vi "I2C Open.vi"(7 "I2C Channel (0)":u8, 8 "Error In":errorcluster, 11 "LINX Resource":T1) -> (0 "Error Out":errorcluster, 3 "LINX Resource":T1)   [LabVIEW 2011, in "LVH-LINX.lvlib"]
doc: "Open the specified I2C channel."
uses:
  LVH-LINX.lvlib
  Private/Type Defs/LINX Ref.ctl
  Private/Type Defs/Platform.ctl
  Private/Type Defs/Interface.ctl
  Private/Device/Type Defs/LINX Device Config.ctl
  Private/Device/Type Defs/TCP Config.ctl
  Private/Device/Type Defs/Channels.ctl
  Private/Type Defs/Peripheral.ctl
  Private/Type Defs/Channel FGV States.ctl
  Private/Device/Device.lvlib
  Private/myRIO/myRIO.lvlib
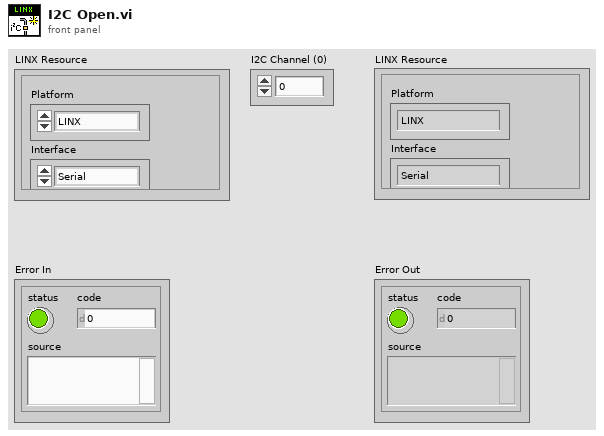
[diagram p1: front panel]
types:
  T1 = typedef "LVH-LINX.lvlib/LINX Ref.ctl" = cluster{"Platform":T2, "Interface":T3, "LINX Device Config":T4}
  T2 = typedef "LVH-LINX.lvlib/Platform.ctl" = enum16{"LINX", "myRIO"}
  T3 = typedef "LVH-LINX.lvlib/Interface.ctl" = enum16{"Serial", "TCP"}
  T4 = typedef "LVH-LINX.lvlib/Device.lvlib/LINX Device Config.ctl" = cluster{"Interface":T3, "COM Port":refnum<visa-resource-name>, "TCP Configuration":T5, "Device Family":u8, "Device ID":u8, "Device Name":string, "TCP Ref":refnum<k5>, "Channels":T6}
  T5 = typedef "LVH-LINX.lvlib/Device.lvlib/TCP Config.ctl" = cluster{"IP Address":string, "Port":u16}
  T6 = typedef "LVH-LINX.lvlib/Channels.ctl" = cluster{"DI Channels":u8[], "DO Channels":u8[], "AI":u8[], "AO":u8[], "PWM":u8[], "QE":u8[], "UART":u8[], "I2C 2":u8[], "SPI":u8[], "CAN":u8[], "AI Ref (V)":dbl, "AO Resolution (Bits)":u8, "AO Ref (V)":dbl}
  T7 = typedef "LVH-LINX.lvlib/Peripheral.ctl" = enum8{"DI", "DO", "AI", "AO", "PWM", "QE", "UART", "I2C", "SPI", "CAN"}
  T8 = typedef "LVH-LINX.lvlib/Channel FGV States.ctl" = enum16{"Initialize", "Get", "Set"}
  T9 = typedef "I2C.lvlib/I2C User Configuration.ctl" = cluster{"I2C Transfer Rate":T10}
  T10 = typedef "I2C.lvlib/I2C Transfer Rate.ctl" = enum16{"Standard Mode (100 kbps)", "Fast Mode (400 kbps)"}
  T11 = typedef "I2C.lvlib/I2C Reference.ctl" = cluster{"myRIO Reference":T12, "I2C Channels Enum":T16, "I2C Configuration":T17}
  T12 = typedef "myRIO Generic Hardware Reference.ctl" = cluster{"myRIO Model":T13, "myRIO Hardware Reference":T14}
  T13 = typedef "Hardware Version Enum.ctl" = enum16{"Unknown", "myRIO-1900", "myRIO-1950"}
  T14 = typedef "myRIO v1.0 Reference.ctl" = cluster{"Generic FPGA Reference":T15, "Allow multiple opens":bool}
  T15 = typedef "Generic FPGA Reference.ctl" = refnum<k20>
  T16 = typedef "I2C Channels Enum.ctl" = enum16{"Not Connected", "A/I2C", "B/I2C"}
  T17 = typedef "I2C.lvlib/I2C Configuration.ctl" = cluster{"I2C Transfer Rate":T10}
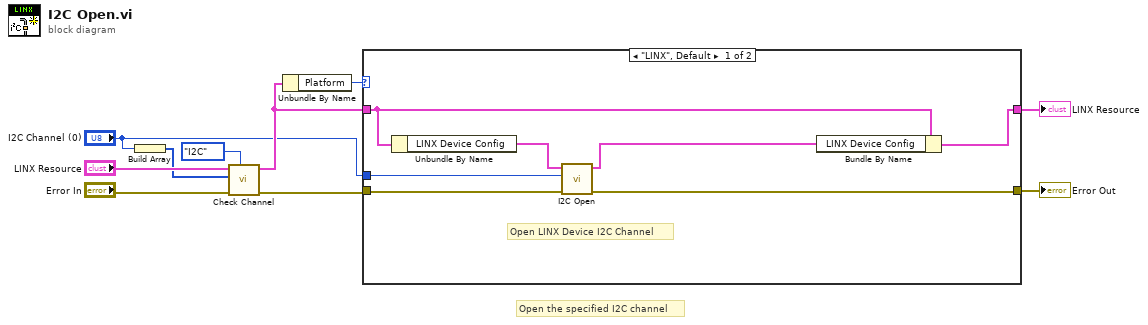
[diagram p0: block diagram]
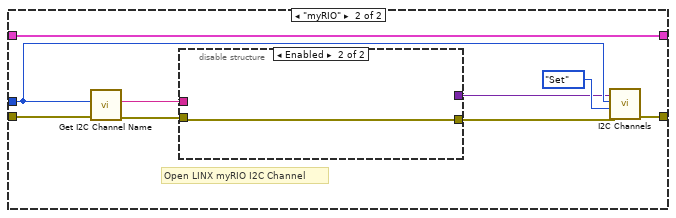
[diagram p2: hidden frame]
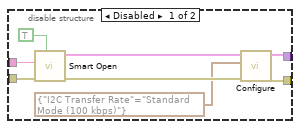
[diagram p3: hidden frame]
diagram:
  # "Open the specified I2C channel"
  n1 = Build Array("I2C Channel (0)") -> (w3:u8[])
  n2 = call "Check Channel.vi"("Peripheral"=Peripheral."I2C", "Error In"="Error In", "Channels"=w3, "LINX Resource"="LINX Resource") -> ("Error Out"=w4:errorcluster, "LINX Resource"=w5:T1)  [unwired: 5 in, 1 out]
  n3 = Unbundle By Name(w5) -> ("Platform"=w10:T2)
  n4 = case shown="\"LINX\", Default" w10 {
    tunnel: w4 -> [w15 w22]
    tunnel: w5 -> [w17 w26]
    tunnel: [w14 w25] -> w9
    tunnel: [w16 w26] -> w8
    tunnel: "I2C Channel (0)" -> [w11 w23]
    frame "LINX", Default {
      # "Open LINX Device I2C Channel"
      n5 = Unbundle By Name(w17) -> ("LINX Device Config"=w12:T4)
      n6 = call "I2C Open.vi"("Error In"=w15, "I2C Channel (0)"=w11, "LINX Device Config"=w12) -> ("Error Out"=w14:errorcluster, "LINX Device Config"=w13:T4)  [unwired: 7 in]
      n7 = Bundle By Name(cluster=w17, "LINX Device Config"=w13) -> (w16:T1)
    }
    frame "myRIO" {
      # "Open LINX myRIO I2C Channel"
      n8 = call "Get I2C Channel Name.vi"("Error In"=w22, "I2C Channel"=w23) -> ("Error Out"=w20:errorcluster, "myRIO I2C Channels"=w19:string)  [unwired: 8 in]
      n9 = disable-structure shown="Enabled" {
        disable-tunnel: [w29 w35] -> w21
        disable-tunnel: w20 -> [w33 w35]
        disable-tunnel: w19 -> [w32 _]
        disable-tunnel: [w30 _] -> w18
        frame Disabled {
          n10 = call <vilib>:"Smart Open.vi"("Allow multiple opens?"=TRUE, "error in (no error)"=w33, "Channel Name"=w32) -> ("error out"=w28:errorcluster, "I2C Ref Out"=w31:T11)  [unwired: 7 in]
          n11 = call <vilib>:"Configure.vi"("error in (no error)"=w28, "I2C User Configuration"=T9 {"I2C Transfer Rate"=enum."Standard Mode (100 kbps)"}, "I2C Ref In"=w31) -> ("error out"=w29:errorcluster, "I2C Ref Out"=w30:T11)  [unwired: 7 in]
        }
        frame Enabled {
        }
      }
      n12 = call "I2C Channels.vi"("Error In"=w21, "Channel State"=Channel_FGV_States."Set", "Channel Number"=w23, "I2C Channel"=w18) -> ("Error Out"=w25:errorcluster)  [unwired: 6 in, 1 out]
    }
  }
  "Error Out" <- w9
  "LINX Resource" <- w8
